vi "Path Crossing Within Limits.vi"(8 "error in (no error)":errorcluster, 9 "Limits":cluster{"Min":i64, "Max":i64}, 10 "Hailstone 2":refnum<class "Hailstone.lvclass">, 11 "Hailstone In":refnum<class "Hailstone.lvclass">) -> (0 "error out":errorcluster, 2 "Crossing?":bool, 3 "Hailstone Out":refnum<class "Hailstone.lvclass">)   [LabVIEW 2021, in "Hailstone.lvclass"]
uses:
  Hailstone.lvclass
  Axis.ctl
  Plane.ctl
  Trace/Trace.lvclass
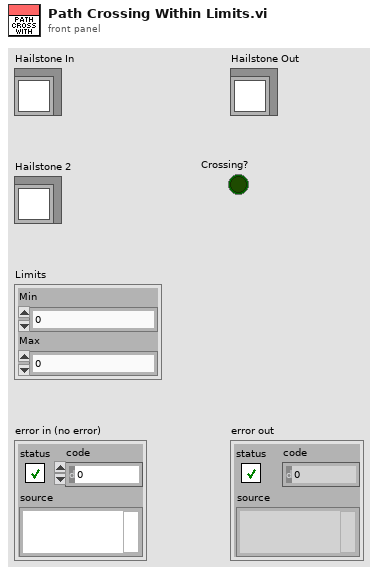
[diagram p1: front panel]
types:
  T1 = typedef "Plane.ctl" = enum16{"XY", "YX"}
  T2 = typedef "Axis.ctl" = enum16{"X", "Y", "Z"}
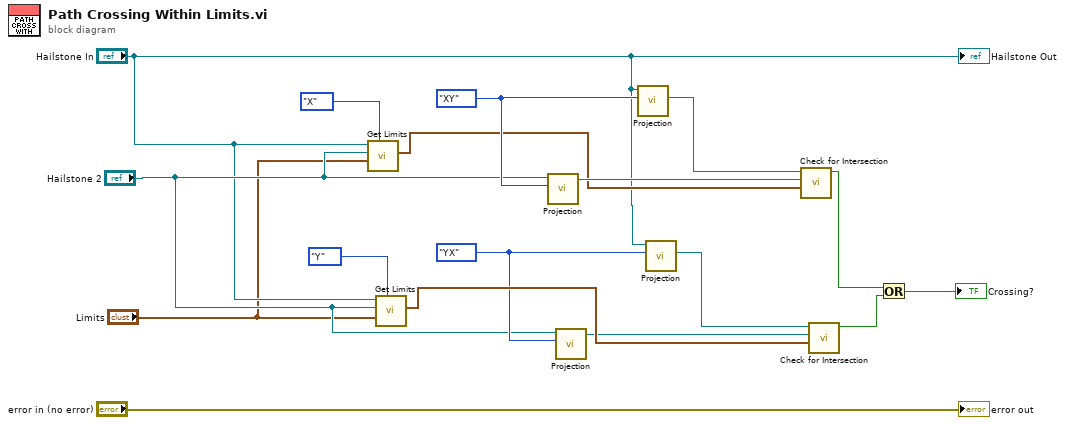
[diagram p0: block diagram]
diagram:
  w6 = Plane."YX" ("Axis")
  w13 = Plane."XY" ("Axis")
  n1 = call "Get Limits.vi"("Axis"=Axis."X", "Limits in"="Limits", "Hailstone 2"="Hailstone 2", "Hailstone in"="Hailstone In") -> ("Limits out"=w11:cluster{"Min":i64, "Max":i64})  [unwired: 7 in]
  n2 = call "Get Limits.vi"("Axis"=Axis."Y", "Limits in"="Limits", "Hailstone 2"="Hailstone 2", "Hailstone in"="Hailstone In") -> ("Limits out"=w10:cluster{"Min":i64, "Max":i64})  [unwired: 7 in]
  n3 = call "Projection.vi"("Axis"=w13, "Hailstone in"="Hailstone 2") -> ("Trace"=w15:refnum<class "Trace.lvclass">)  [unwired: 9 in]
  n4 = call "Projection.vi"("Axis"=w6, "Hailstone in"="Hailstone 2") -> ("Trace"=w7:refnum<class "Trace.lvclass">)  [unwired: 9 in]
  n5 = call "Projection.vi"("Axis"=w13, "Hailstone in"="Hailstone In") -> ("Trace"=w14:refnum<class "Trace.lvclass">)  [unwired: 9 in]
  n6 = call "Projection.vi"("Axis"=w6, "Hailstone in"="Hailstone In") -> ("Trace"=w8:refnum<class "Trace.lvclass">)  [unwired: 9 in]
  n7 = call "Check for Intersection.vi"("Limits in"=w11, "Hailstone 2"=w15, "Trace In"=w14) -> ("Boolean"=w16:bool)  [unwired: 8 in]
  n8 = call "Check for Intersection.vi"("Limits in"=w10, "Hailstone 2"=w7, "Trace In"=w8) -> ("Boolean"=w2:bool)  [unwired: 8 in]
  n9 = Or(x=w16, y=w2) -> (x .or. y?=→"Crossing?":bool)
  "error out" <- "error in (no error)"
  "Hailstone Out" <- "Hailstone In"
